vi "Parent.vi"(10 "error in (no error)":errorcluster, 11 "Config Element in":refnum<class "Config Element.lvclass">) -> (2 "error out":errorcluster, 3 "Parent":refnum<class "Config Element.lvclass">)   [LabVIEW 2020, in "CDM-Config.lvlib" / "Config Element.lvclass"]
uses:
  Config Element.lvclass
  Config Manager/Config Manager.lvclass
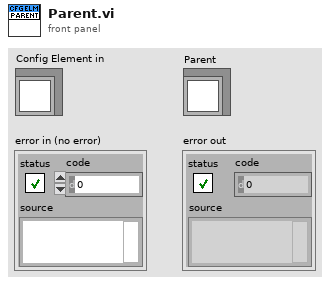
[diagram p1: front panel]
types:
  T1 = typedef "CDM-Config.lvlib/Config Element.lvclass/Ref Data.ctl" = cluster{"Node Info":T2, "Owner":refnum<class>, "Changed":bool, "Name":string, "Value":string, "Meta Data":T3[]}
  T2 = typedef "CDM-Config.lvlib/Node Info.ctl" = cluster{"Index":i32, "Parent":i32, "Children":i32[]}
  T3 = typedef "CDM-Config.lvlib/Meta Data.ctl" = cluster{"Name":string, "Value":string}
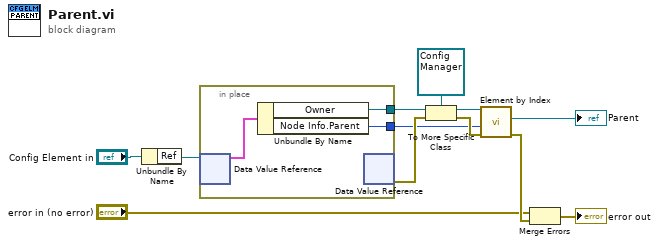
[diagram p0: block diagram]
diagram:
  n1 = Unbundle By Name("Config Element in") -> ("Ref"=w11:refnum<data-value>)
  n2 = in-place {
    in-place-border: [w14] -> w6
    in-place-border: [w13] -> w10
    n3 = in-place-dvr #1(w11) -> (w15:T1)  [unwired: 1 out]
    n4 = Unbundle By Name(w15) -> ("Owner"=w13:refnum<class>, "Node Info.Parent"=w14:i32)
    n5 = in-place-dvr #1() -> (w9:errorcluster)  [unwired: 1 in, 1 out]
  }
  n6 = To More Specific Class(target class=refnum<class "Config Manager.lvclass"> refnum ("CDM-Config.lvlib:Config Manager.lvclass"), reference=w10, error in=w9) -> (specific class reference=w7:refnum<class "Config Manager.lvclass">, error out=w12:errorcluster)
  n7 = call "Element by Index.vi"("error in (no error)"=w12, "Index"=w6, "Config Manager in"=w7) -> ("error out"=w5:errorcluster, "Element"=→"Parent":refnum<class "Config Element.lvclass">)  [unwired: 6 in, 1 out]
  n8 = Merge Errors("error in (no error)", w5) -> (→"error out":errorcluster)
